vi "Destroy Event.vi"(8 "error in (no error)":errorcluster, 11 "Messaging in":refnum<class "Messaging.lvclass">) -> (0 "error out":errorcluster, 3 "Messaging out":refnum<class "Messaging.lvclass">)   [LabVIEW 2023, in "Messaging.lvclass"]
uses:
  Messaging.lvclass
  Messaging.lvclass/Messaging.ctl
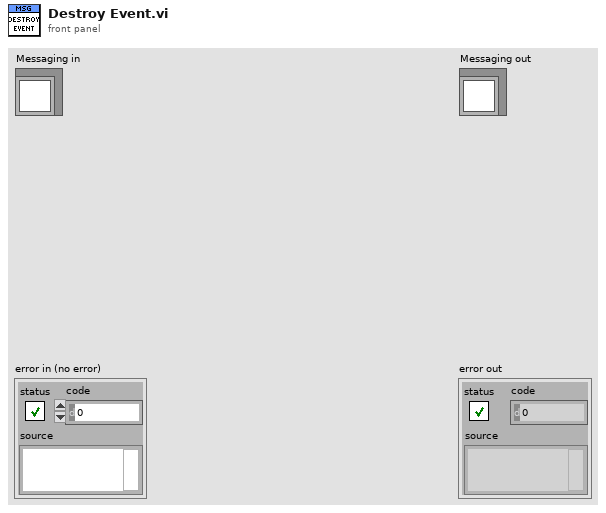
[diagram p1: front panel]
types:
  T1 = typedef "Msg.Event.Ref.ctl" = refnum<user-event>
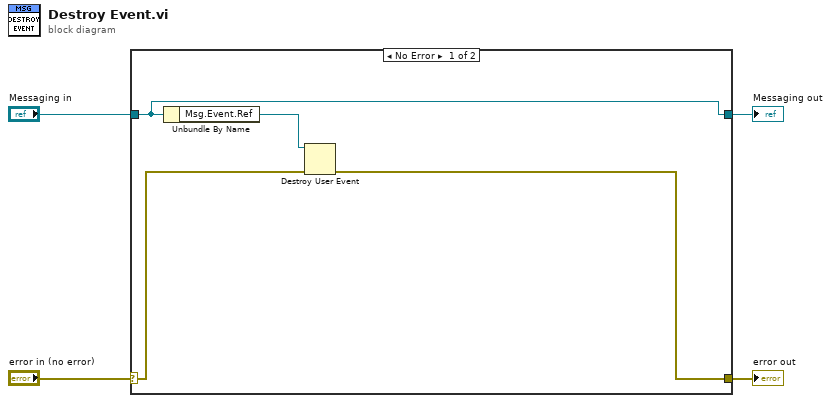
[diagram p0: block diagram]
diagram:
  n1 = case shown="No Error" "error in (no error)" {
    selector: "error in (no error)" -> [w6 w10]
    tunnel: [w8 w10] -> w3
    tunnel: [w5 w9] -> w1
    tunnel: "Messaging in" -> [w5 w9]
    frame No Error {
      n2 = Unbundle By Name(w5) -> ("Msg.Event.Ref"=w7:T1)
      n3 = Destroy User Event(user event=w7, error in=w6) -> (error out=w8:errorcluster)
    }
    frame Error {
    }
  }
  "error out" <- w3
  "Messaging out" <- w1
